vi "liblinear_add_node_padding.vi"(8 "error in (no error)":errorcluster, 11 "Nodes":T1[](array[typedef])) -> (0 "error out":errorcluster, 3 "Padded nodes":T2[](array[typedef]))   [LabVIEW 2014]
uses:
  Controls/liblinear_node_padded.ctl
  Controls/liblinear_node.ctl
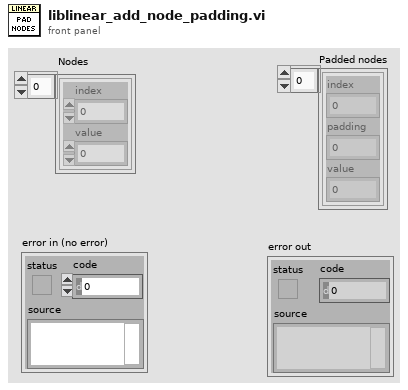
[diagram p1: front panel]
types:
  T1 = typedef "liblinear_node.ctl" = cluster{"index":i32, "value":dbl}
  T2 = typedef "liblinear_node_padded.ctl" = cluster{"index":i32, "padding":i32, "value":dbl}
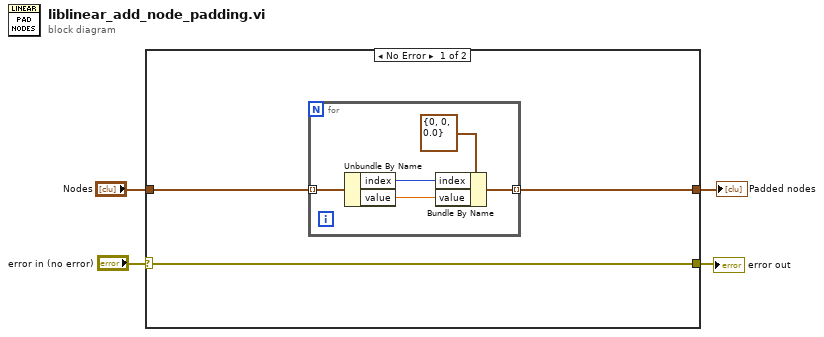
[diagram p0: block diagram]
diagram:
  n1 = case shown="No Error" "error in (no error)" {
    selector: "error in (no error)" -> [w7 w13]
    tunnel: [w7 w13] -> w4
    tunnel: "Nodes" -> [w6 _]
    tunnel: [w5 _] -> w1
    frame No Error {
      n2 = for {
        tunnel: w6 -> [w12] mode=indexing
        tunnel: [w8] -> w5 mode=indexing
        n3 = Unbundle By Name(w12) -> ("index"=w11:i32, "value"=w10:dbl)
        n4 = Bundle By Name(cluster=T2 {"index"=0, "padding"=0, "value"=0.0} ("feature_node"), "index"=w11, "value"=w10) -> (w8:T2)
      }
    }
    frame Error {
    }
  }
  "error out" <- w4
  "Padded nodes" <- w1
